vi "数据流观察.vi"() -> ()   [LabVIEW 2011]
panel:
  in  "停止":bool
  out "数值 2":dbl
  in  "d":dbl
  in  "c":dbl
  in  "b":dbl
  in  "a":dbl
  out "数值 1":dbl
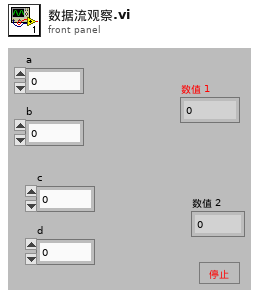
[diagram p1: front panel]
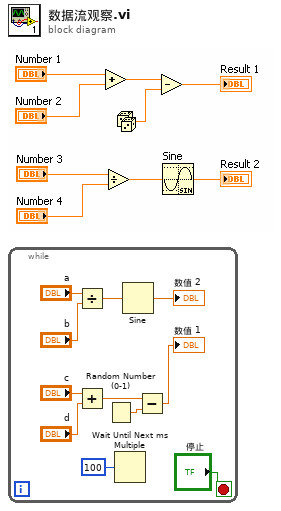
[diagram p0: block diagram]
diagram:
  n1 = while {
    stop <- "停止" stop-if-true
    n2 = Divide(x="a", y="b") -> (x/y=w7:dbl)
    n3 = Add(x="c", y="d") -> (x+y=w11:dbl)
    n4 = Random Number (0-1)() -> (number: 0 to 1=w10:dbl)
    n5 = Wait Until Next ms Multiple(millisecond multiple=u32 100 ("毫秒倍数")) -> ()  [unwired: 1 out]
    n6 = Sine(x=w7) -> (sin(x)=→"数值 2":dbl)
    n7 = Subtract(x=w11, y=w10) -> (x-y=→"数值 1":dbl)
  }
